vi "escal.vi"(9 "Escala":i32, 10 "image data":T1, 11 "24-bit pixmap in":u32[][](array[numeric])) -> (3 "24-bit pixmap out":u32[][](array[numeric]))   [LabVIEW 2019]
uses:
  <vilib>/picture/picture.llb/imagedata.ctl
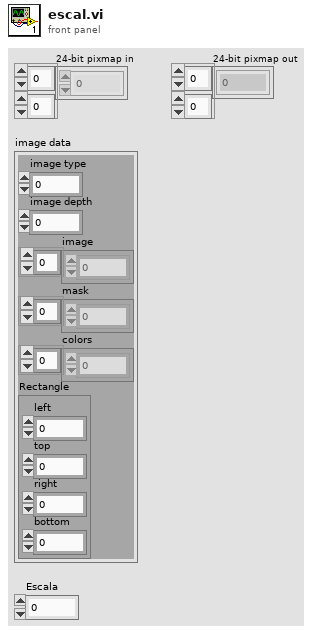
[diagram p1: front panel]
types:
  T1 = typedef "imagedata.ctl" = cluster{"image type":i32, "image depth":i32, "image":u8[], "mask":u8[], "colors":u32[], "Rectangle":cluster{"left":i16, "top":i16, "right":i16, "bottom":i16}}
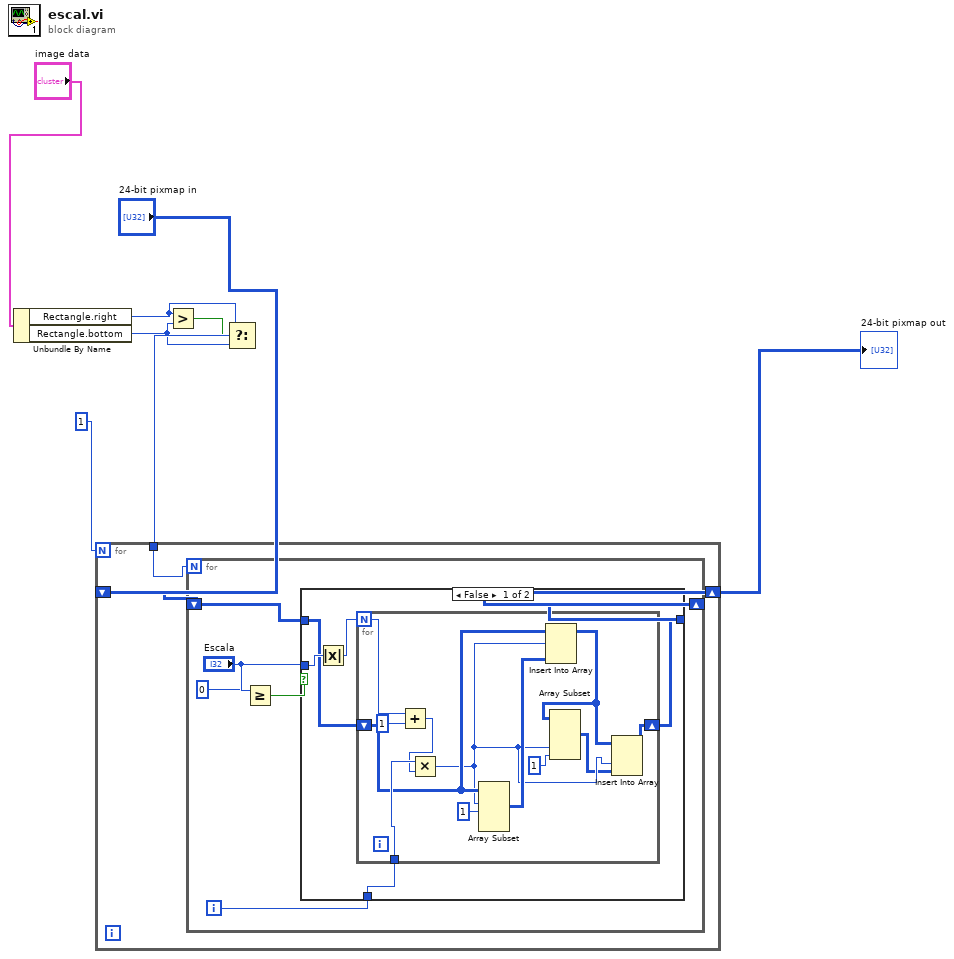
[diagram p0: block diagram]
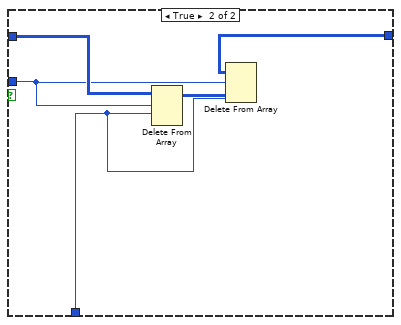
[diagram p2: hidden frame]
diagram:
  n1 = Unbundle By Name("image data") -> ("Rectangle.right"=w5:i16, "Rectangle.bottom"=w6:i16)
  n2 = Greater?(x=w5, y=w6) -> (0:w4:bool)
  n3 = Select(t=w5, s=w4, f=w6) -> (s? t:f=w7:i16)
  n4 = for {
    N: 1 -> [_]
    shift-right: [w10] -> w3
    shift-left: "24-bit pixmap in" -> [w11]
    tunnel: w7 -> [w9]
    n5 = for {
      N: w9 -> [_]
      shift-right: [w16] -> w10
      shift-left: w11 -> [w17]
      i -> [w12]
      n6 = Greater Or Equal?(x="Escala", y=0) -> (x >= y?=w13:bool)
      n7 = case shown="False" w13 {
        tunnel: w17 -> [w18 w39]
        tunnel: [w19 w37] -> w16
        tunnel: "Escala" -> [w22 w36]
        tunnel: w12 -> [w20 w35]
        frame False {
          n8 = Absolute Value(x=w22) -> (abs(x)=w21:i32)
          n9 = for {
            N: w21 -> [w32]
            tunnel: w20 -> [w33]
            shift-right: [w24] -> w19
            shift-left: w18 -> [w28]
            n10 = Add(x=w32, y=1) -> (x+y=w30:i32)
            n11 = Multiply(x=w33, y=w30) -> (x*y=w26:i32)
            n12 = Array Subset(array=w28, index (row)=w26, length (row)=1 ("length")) -> (w34:u32[][])  [unwired: 2 in]
            n13 = Insert Into Array(array=w28, index (row)=w26, new element=w34) -> (w23:u32[][])  [unwired: 1 in]
            n14 = Array Subset(array=w23, index (col)=w26, length (col)=1 ("length")) -> (w25:u32[][])  [unwired: 2 in]
            n15 = Insert Into Array(array=w23, index (col)=w26, new element=w25) -> (w24:u32[][])  [unwired: 1 in]
          }
        }
        frame True {
          n16 = Delete From Array(array=w39, length=w36, index (row)=w35) -> (array with subset deleted=w38:u32[][])  [unwired: 1 in, 1 out]
          n17 = Delete From Array(array=w38, length=w36, index (col)=w35) -> (array with subset deleted=w37:u32[][])  [unwired: 1 in, 1 out]
        }
      }
    }
  }
  "24-bit pixmap out" <- w3
